vi "Launch Nested.vi"(8 "error in":errorcluster, 9 "ID":string, 10 "Nested Actor":refnum<class "Actor.lvclass">, 11 "SuperActor in":refnum<class "SuperActor.lvclass">) -> (0 "error out":errorcluster, 2 "Launch Successful?":bool, 3 "SuperActor out":refnum<class "SuperActor.lvclass">)   [LabVIEW 2016, in "SuperActor.lvlib" / "SuperActor.lvclass"]
uses:
  SuperActor.lvclass
  C:/Program Files (x86)/National Instruments/LabVIEW 2016/vi.lib/ActorFramework/Actor/Actor.lvclass
  <vilib>/ActorFramework/Actor/Actor.lvclass
  SuperActor.lvclass/SuperActor.ctl
  Session APIs/Session Log/System Log.lvclass
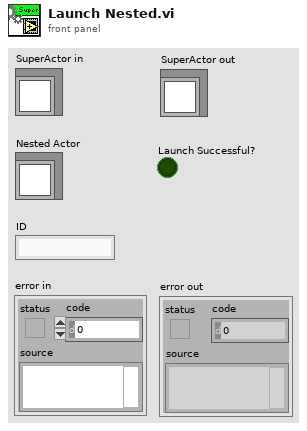
[diagram p1: front panel]
types:
  T1 = typedef "Session - Root.lvclass/Session Handle.ctl" = refnum<data-value>
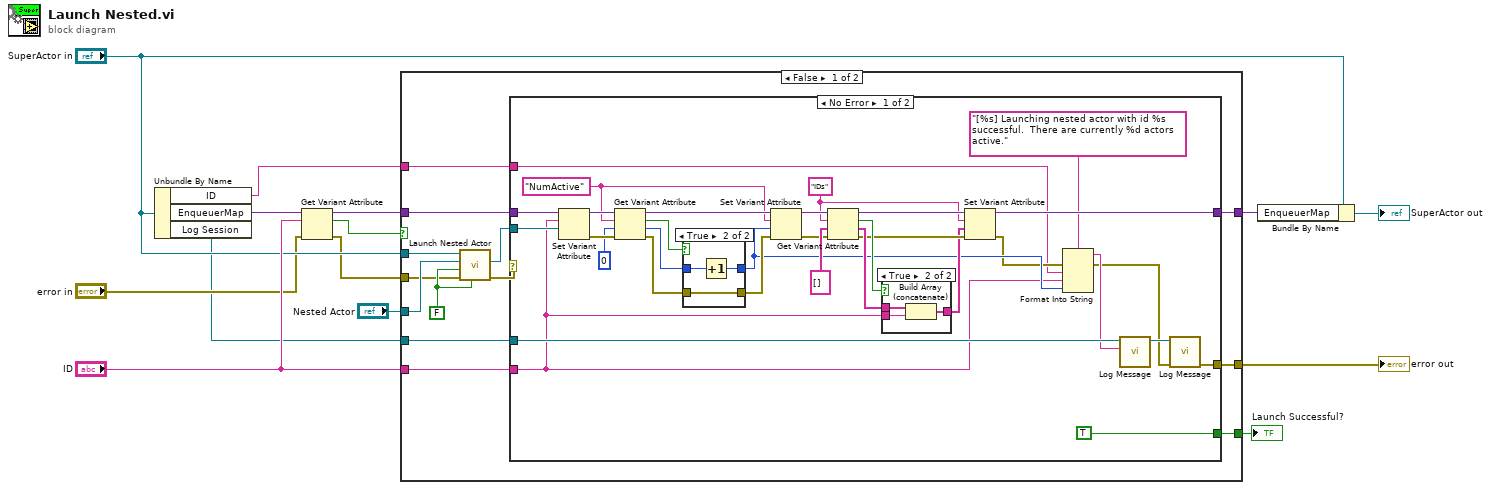
[diagram p0: block diagram]
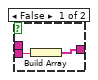
[diagram p2: hidden frame]
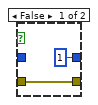
[diagram p3: hidden frame]
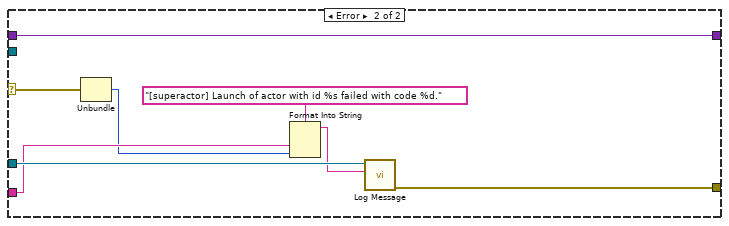
[diagram p4: hidden frame]
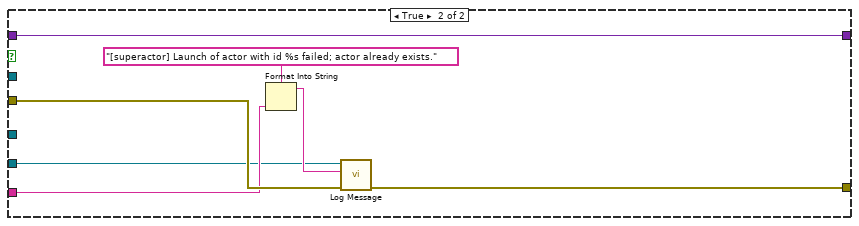
[diagram p5: hidden frame]
diagram:
  n1 = Unbundle By Name("SuperActor in") -> ("ID"=w2:string, "EnqueuerMap"=w13:variant, "Log Session"=w3:T1)
  n2 = Get Variant Attribute(Variant=w13, name="ID", error in="error in") -> (duplicate Variant=w11:variant, found=w12:bool, error out=w6:errorcluster)  [unwired: 1 in, 1 out]
  n3 = case shown="False" w12 {
    tunnel: "SuperActor in" -> [w27 _]
    tunnel: "Nested Actor" -> [w26 _]
    tunnel: w11 -> [w22 w84]
    tunnel: "ID" -> [w21 w79]
    tunnel: [w20 w84] -> w8
    tunnel: w6 -> [w19 w80]
    tunnel: [w18 w81] -> w5
    tunnel: w3 -> [w17 w78]
    tunnel: w2 -> [w16 _]
    tunnel: [w15 _] -> w1
    frame False {
      w25 = FALSE ("Auto-stop? (T)")
      n4 = call <vilib>:"Launch Nested Actor.vi"("Open Actor Core front panel? (F)"=w25, "error in (no error)"=w19, "Auto-stop? (T)"=w25, "Nested Actor"=w26, "Caller Actor in"=w27) -> ("error out"=w24:errorcluster, "Nested Actor's Enqueuer"=w23:refnum<class "Message Enqueuer.lvclass">)  [unwired: 4 in, 1 out]
      n5 = case shown="No Error" w24 {
        selector: w24 -> [_ w74]
        tunnel: w23 -> [w58 _]
        tunnel: w22 -> [w59 w70]
        tunnel: w21 -> [w30 w75]
        tunnel: [w39 w70] -> w20
        tunnel: w17 -> [w38 w77]
        tunnel: [w33 w71] -> w18
        tunnel: w16 -> [w29 _]
        tunnel: [TRUE _] -> w15
        frame No Error {
          w44 = "IDs" ("name")
          w41 = "NumActive" ("name")
          n6 = Set Variant Attribute(Variant=w59, name=w30, value=w58) -> (Variant out=w43:variant, error out=w42:errorcluster)  [unwired: 1 in, 1 out]
          n7 = Get Variant Attribute(Variant=w43, name=w41, default value (empty Variant)=i16 0 ("unsigned 8bit integer"), error in=w42) -> (duplicate Variant=w56:variant, found=w55:bool, value=w57:i16, error out=w54:errorcluster)
          n8 = case shown="True" w55 {
            tunnel: w57 -> [_ w67]
            tunnel: [i16 1 w69] -> w36
            tunnel: w54 -> [w65 w68]
            tunnel: [w65 w68] -> w53
            frame False {
            }
            frame True {
              n9 = Increment(x=w67) -> (x+1=w69:i16)
            }
          }
          n10 = Set Variant Attribute(Variant=w56, name=w41, value=w36, error in=w53) -> (Variant out=w52:variant, error out=w50:errorcluster)  [unwired: 1 out]
          n11 = Get Variant Attribute(Variant=w52, name=w44, default value (empty Variant)=string[] [], error in=w50) -> (duplicate Variant=w47:variant, found=w49:bool, value=w48:string[], error out=w46:errorcluster)
          n12 = case shown="True" w49 {
            tunnel: w48 -> [_ w64]
            tunnel: w30 -> [w61 w63]
            tunnel: [w60 w62] -> w45
            frame False {
              n13 = Build Array(w61) -> (w60:string[])
            }
            frame True {
              n14 = Build Array (concatenate)(w64, w63) -> (w62:string[])
            }
          }
          n15 = Set Variant Attribute(Variant=w47, name=w44, value=w45, error in=w46) -> (Variant out=w39:variant, error out=w32:errorcluster)  [unwired: 1 out]
          n16 = Format Into String(format string="[%s] Launching nested actor with id %s successful.  There are currently %d actors active.", error in=w32, w29, w30, w36) -> (resulting string=w35:string, error out=w31:errorcluster)  [unwired: 1 in]
          n17 = call "Log Message.vi"("MSG In"=w35, "session in"=w38) -> ("session out"=w34:T1)  [unwired: 8 in, 1 out]
          n18 = call "Log Message.vi"("error in"=w31, "session in"=w34) -> ("error out"=w33:errorcluster)  [unwired: 8 in, 1 out]
        }
        frame Error {
          n19 = Unbundle(w74) -> ("code"=w73:i32)  [unwired: 2 out]
          n20 = Format Into String(format string="[superactor] Launch of actor with id %s failed with code %d.", w75, w73) -> (resulting string=w72:string)  [unwired: 2 in, 1 out]
          n21 = call "Log Message.vi"("MSG In"=w72, "session in"=w77) -> ("error out"=w71:errorcluster)  [unwired: 8 in, 1 out]
        }
      }
    }
    frame True {
      n22 = Format Into String(format string="[superactor] Launch of actor with id %s failed; actor already exists.", w79) -> (resulting string=w82:string)  [unwired: 2 in, 1 out]
      n23 = call "Log Message.vi"("error in"=w80, "MSG In"=w82, "session in"=w78) -> ("error out"=w81:errorcluster)  [unwired: 7 in, 1 out]
    }
  }
  "error out" <- w5
  "Launch Successful?" <- w1
  n24 = Bundle By Name(cluster="SuperActor in", "EnqueuerMap"=w8) -> (→"SuperActor out":refnum<class "SuperActor.lvclass">)
